vi "解析S2文件.vi"() -> ()   [LabVIEW 2017]
panel:
  out "段地址":u32[](array[numeric]) format="%6x"
  out "输出数组-第一行":i32[][](array[numeric]) format="%02x"
  out "发送数据组":u32[][][](array[numeric]) format="%02x"
  out "数组头-每段":u32[][](array[numeric]) format="%x"
  out "连续数组-中-每小块":u32[][][](array[numeric]) format="%02x"
  out "数据数组2":u32[][](array[numeric]) format="%02x"
  out "地址有间隔":i32[](array[numeric])
  out "段数":i32
  out "数据数组":string[](array[string])
  out "每行字符数":i32[](array[numeric])
  out "地址数组":u32[](array[numeric]) format="%06x"
  in  "停止":bool
  out "行数":i32
  out "数组":string[](array[string])
  # "段尾"
  # "行数"
  # "每行字符"
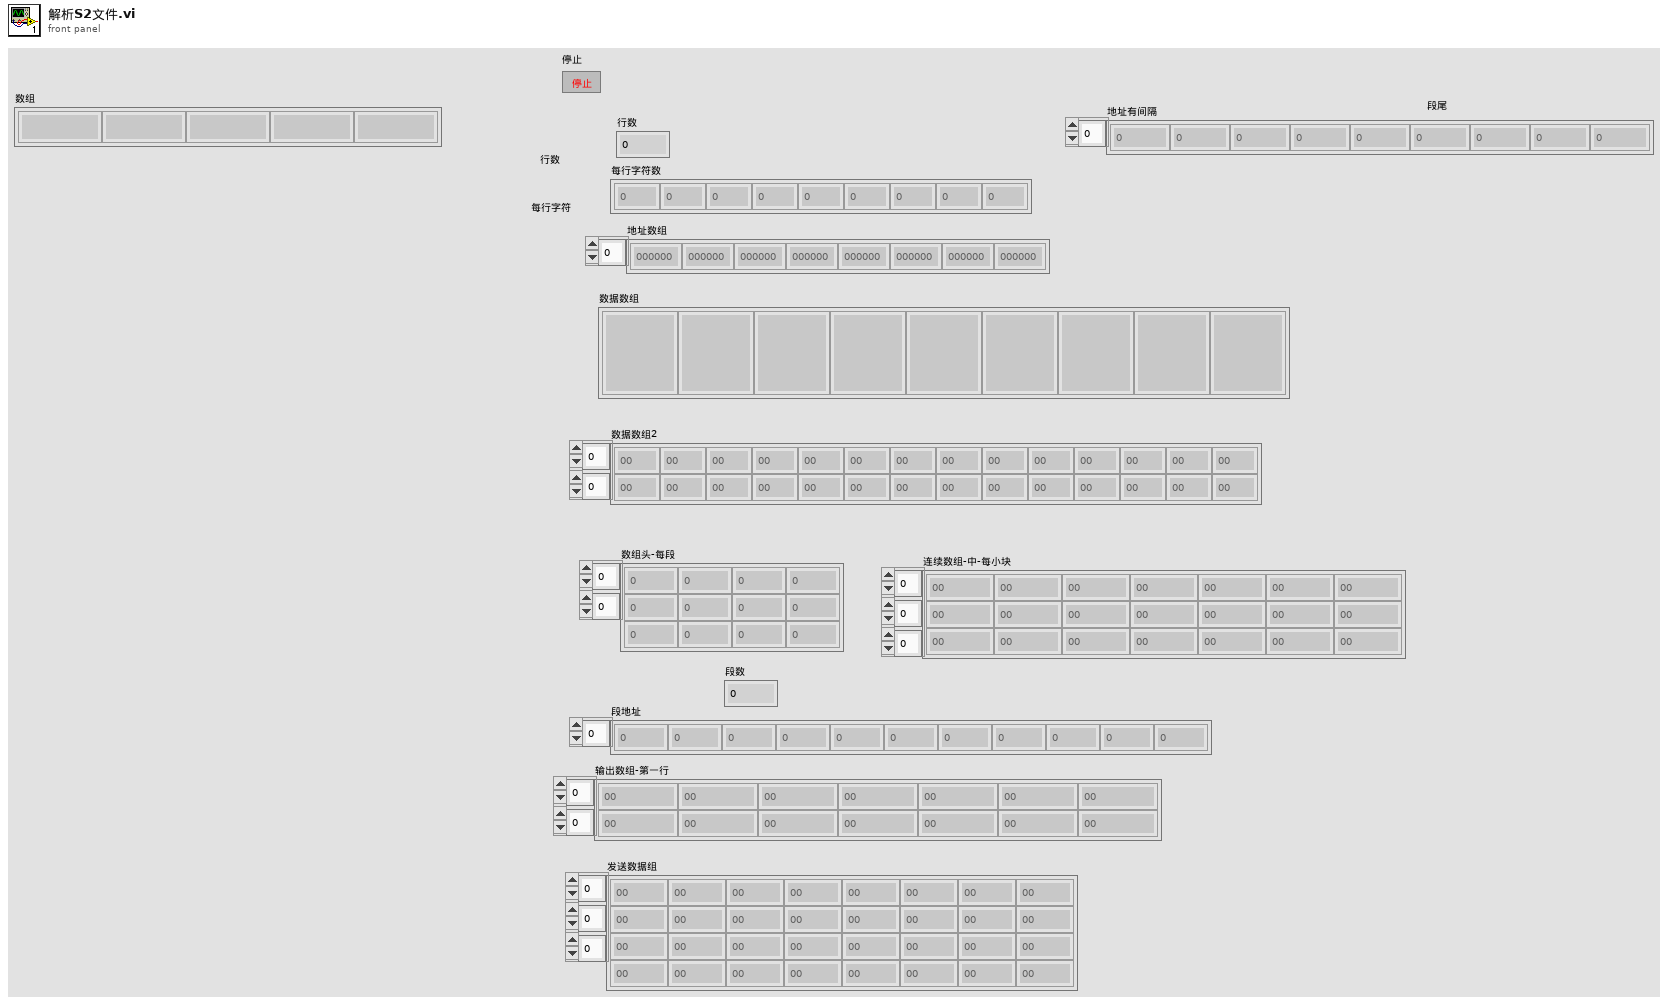
[diagram p1: front panel]
types:
  T1 = enum16{"open", "replace", "create", "open or create", "replace or create", "replace or create with confirmation"}
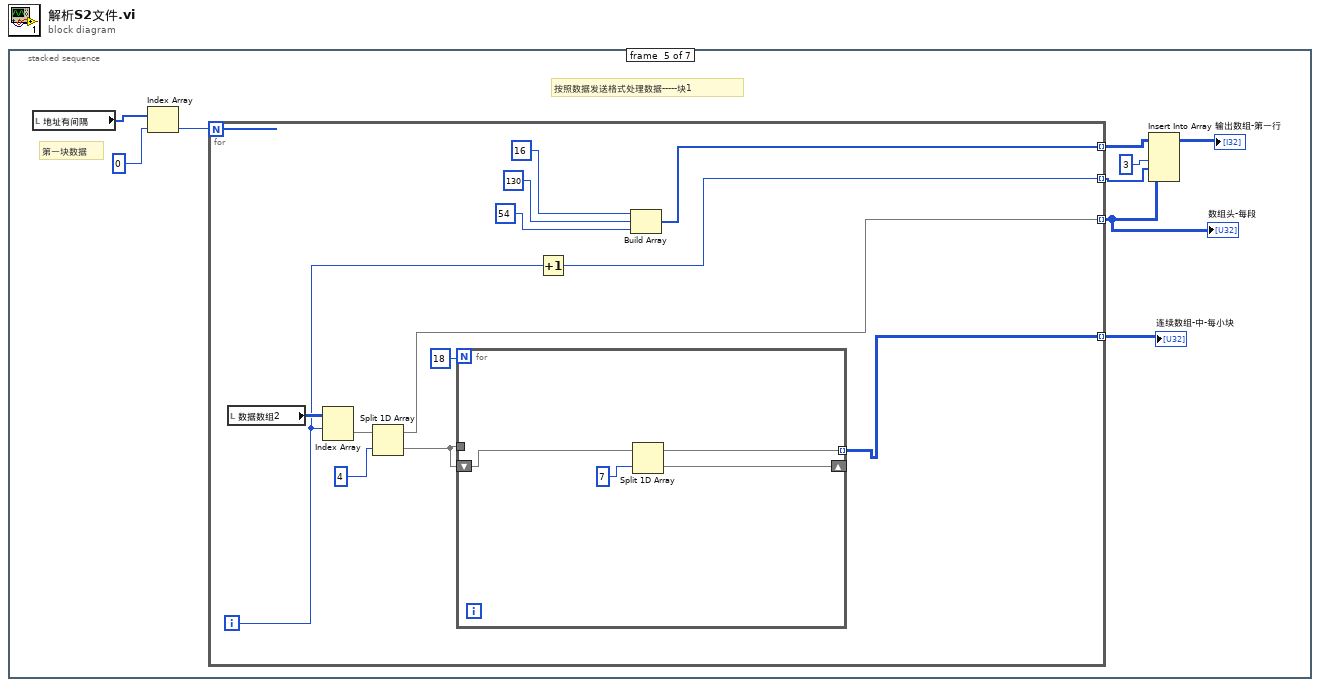
[diagram p0: block diagram]
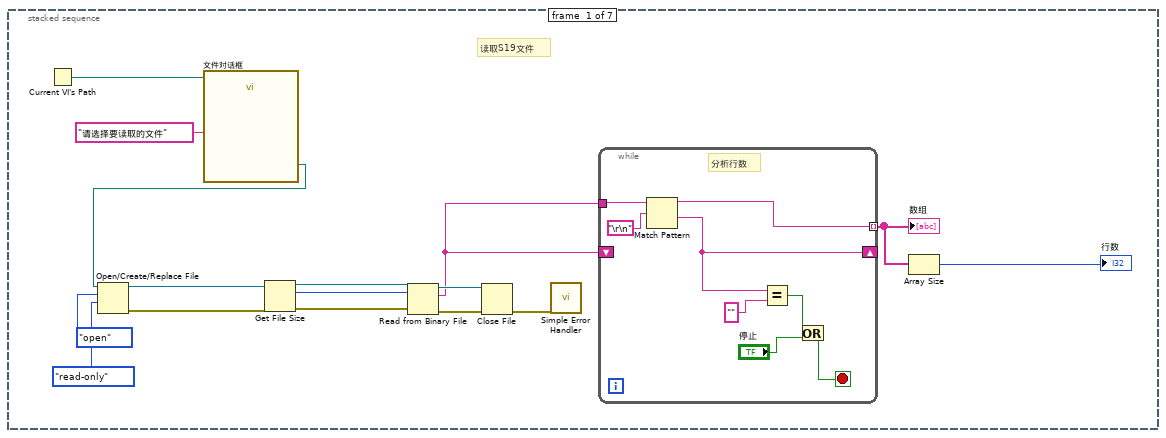
[diagram p2: hidden frame]
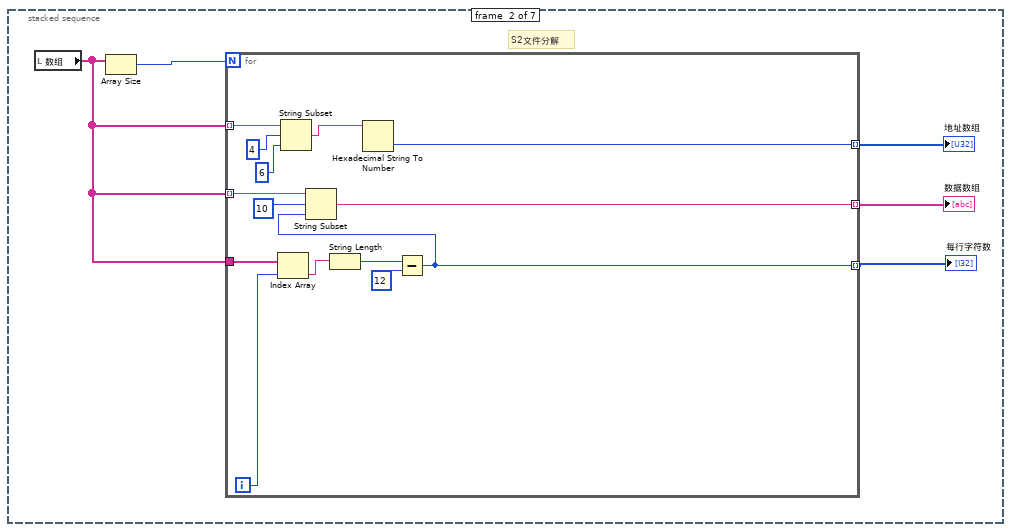
[diagram p3: hidden frame]
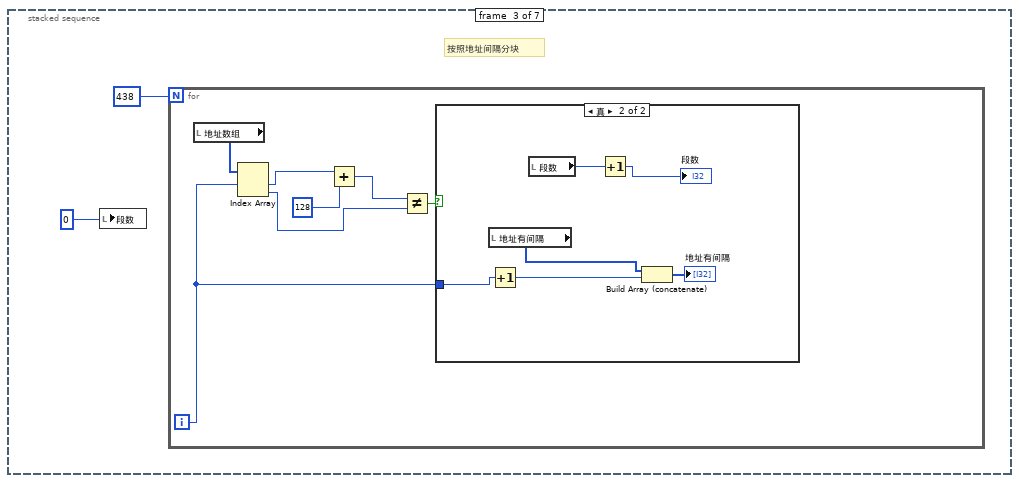
[diagram p4: hidden frame]
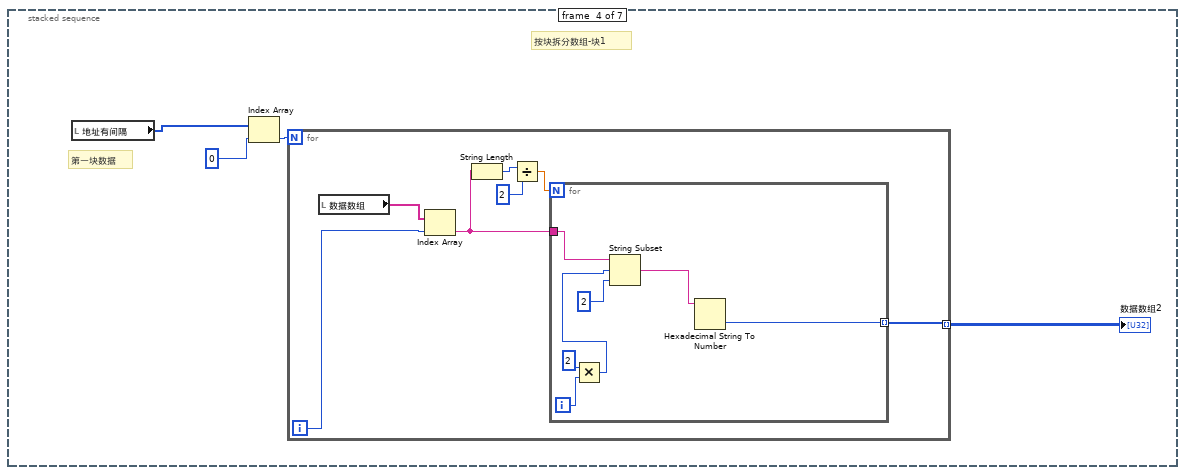
[diagram p6: hidden frame]
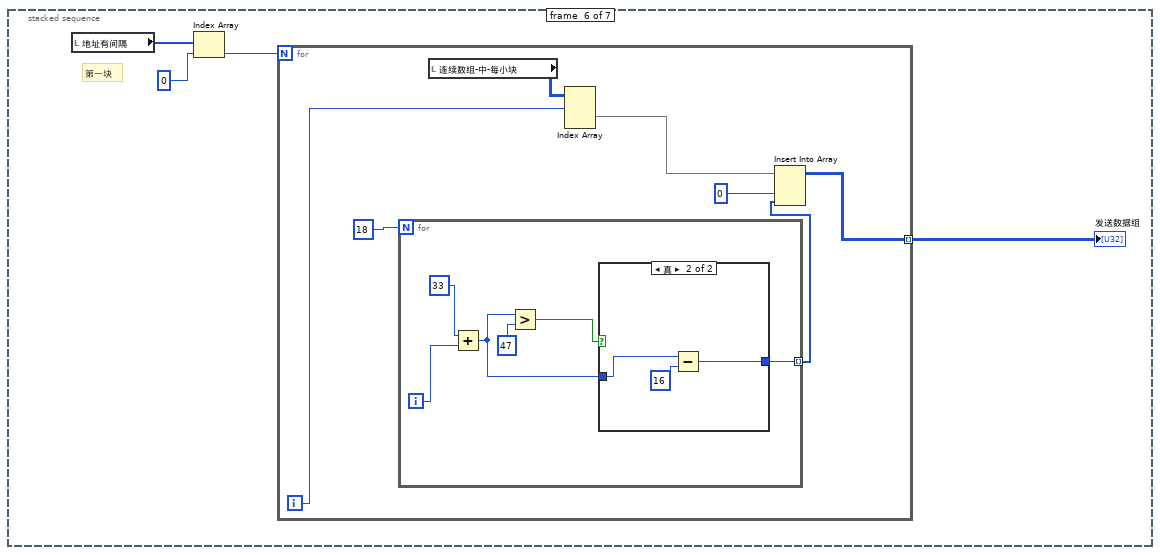
[diagram p7: hidden frame]
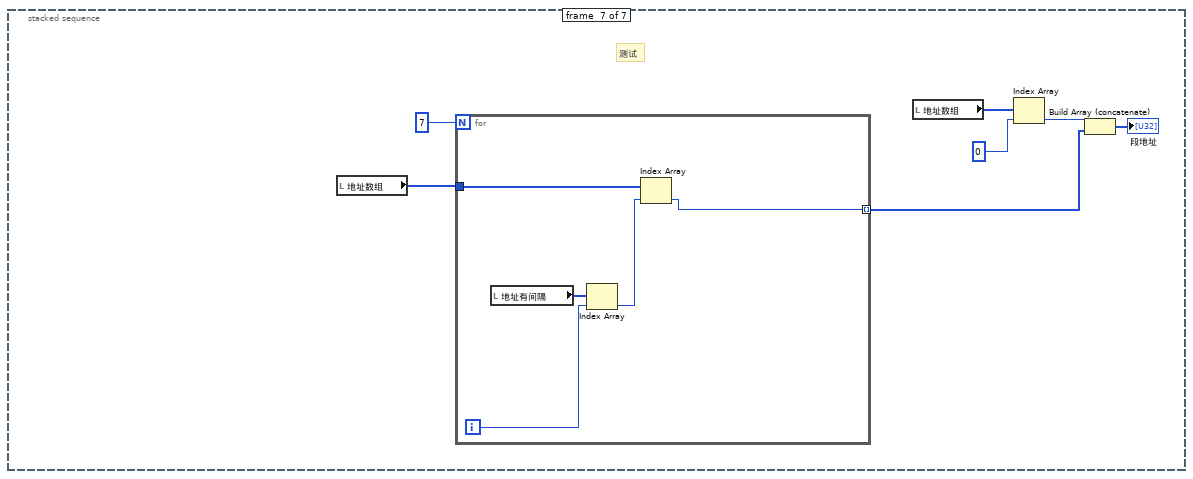
[diagram p9: hidden frame]
diagram:
  n1 = stacked-sequence {
    frame #0 {
      # "读取S19文件"
      n2 = Current VI's Path() -> (path=w5:path)
      n3 = call "文件对话框"("start path"=w5, "prompt"="请选择要读取的文件") -> ("selected path"=w15:path)  [unwired: 10 in, 3 out]
      n4 = Open/Create/Replace File(file path (use dialog)=w15, operation (0:open)=T1."open", access (0:read/write)=enum16{"read/write", "read-only", "write-only"}."read-only") -> (refnum out=w6:refnum<file>, error out=w11:errorcluster)  [unwired: 3 in, 1 out]
      n5 = Get File Size(file=w6, error in=w11) -> (refnum out=w14:refnum<file>, size (in bytes)=w7:i64, 0:w10:errorcluster)
      n6 = Read from Binary File(8:w10, 10:w7, 11:w14) -> (0:w9:errorcluster, 2:w2:string, 3:w16:refnum<file>)  [unwired: 3 in, 1 out]
      n7 = Close File(refnum=w16, error in=w9) -> (error out=w8:errorcluster)  [unwired: 1 out]
      n8 = call <vilib>:"Simple Error Handler.vi"("error in (no error)"=w8) -> ()  [unwired: 4 in, 5 out]
      n9 = while "While循环" {
        tunnel: w2 -> [_]
        tunnel: [w19] -> w1 mode=indexing
        shift-right: [w18] -> _
        shift-left: w2 -> [w17]
        stop <- w22 stop-if-true
        # "分析行数"
        n10 = Match Pattern(string=w17, regular expression="\r\n") -> (before substring=w19:string, after substring=w18:string)  [unwired: 1 in, 2 out]
        n11 = Equal?(x=w18, y="") -> (x = y?=w23:bool)
        n12 = Or(x=w23, y="停止") -> (x .or. y?=w22:bool)
      }
      "数组" <- w1
      n13 = Array Size(array=w1) -> (size(s)=→"行数":i32)
    }
    frame #1 {
      # "S2文件分解"
      n14 = local read "数组"() -> (w27:string[])
      n15 = Array Size(array=w27) -> (size(s)=w25:i32)
      n16 = for {
        N: w25 -> [_]
        tunnel: w27 -> [w43] mode=indexing
        tunnel: [w39] -> w29 mode=indexing
        tunnel: w27 -> [w31]
        tunnel: [w30] -> w28 mode=indexing
        tunnel: w27 -> [w35] mode=indexing
        tunnel: [w33] -> w26 mode=indexing
        i -> [w32]
        n17 = Index Array(array=w31, index=w32) -> (element=w38:string)
        n18 = String Subset(string=w43, offset (0)=4, length (rest)=6) -> (substring=w40:string)
        n19 = String Length(string=w38) -> (length=w37:i32)
        n20 = Hexadecimal String To Number(string=w40) -> (number=w39:u32)  [unwired: 2 in, 1 out]
        n21 = Subtract(x=w37, y=12) -> (x-y=w30:i32)
        n22 = String Subset(string=w35, offset (0)=10, length (rest)=w30) -> (substring=w33:string)
      }
      "地址数组" <- w29
      "每行字符数" <- w28
      "数据数组" <- w26
    }
    frame #2 {
      # "按照地址间隔分块"
      n23 = local write "段数"(0) -> ()
      n24 = for {
        N: 438 -> [_]
        i -> [w49]
        n25 = local read "地址数组"() -> (w50:u32[])
        n26 = Index Array(array=w50, index #1=w49) -> (element #1=w51:u32, element #2=w46:u32)  [unwired: 1 in]
        n27 = Add(x=w51, y=u32 128) -> (x+y=w47:u32)
        n28 = Not Equal?(x=w47, y=w46) -> (x != y?=w48:bool)
        n29 = case shown="真" w48 {
          tunnel: w49 -> [_ w54]
          frame False {
          }
          frame True {
            n30 = local read "地址有间隔"() -> (w55:i32[])
            n31 = Increment(x=w54) -> (x+1=w53:i32)
            n32 = local read "段数"() -> (w58:i32)
            n33 = Increment(x=w58) -> (x+1=→"段数":i32)
            n34 = Build Array (concatenate)(w55, w53) -> (→"地址有间隔":i32[])
          }
        }
      }
    }
    frame #3 {
      # "第一块数据"
      # "按块拆分数组-块1"
      n35 = local read "地址有间隔"() -> (w60:i32[])
      n36 = Index Array(array=w60, index=0) -> (element=w61:i32)
      n37 = for {
        N: w61 -> [_]
        tunnel: [w64] -> w62 mode=indexing
        i -> [w63]
        n38 = local read "数据数组"() -> (w66:string[])
        n39 = Index Array(array=w66, index=w63) -> (element=w67:string)
        n40 = String Length(string=w67) -> (length=w68:i32)
        n41 = Divide(x=w68, y=2) -> (x/y=w69:dbl)
        n42 = for {
          N: w69 -> [_]
          tunnel: w67 -> [w76]
          tunnel: [w74] -> w64 mode=indexing
          i -> [w73]
          n43 = Multiply(x=2, y=w73) -> (x*y=w72:i32)
          n44 = String Subset(string=w76, offset (0)=w72, length (rest)=2) -> (substring=w75:string)
          n45 = Hexadecimal String To Number(string=w75) -> (number=w74:u32)  [unwired: 2 in, 1 out]
        }
      }
      "数据数组2" <- w62
    }
    frame #4 {
      # "第一块数据"
      # "按照数据发送格式处理数据-----块1"
      n46 = local read "地址有间隔"() -> (w85:i32[])
      n47 = Index Array(array=w85, index=0) -> (element=w83:i32)
      n48 = for {
        N: w83 -> [_]
        tunnel: [w93] -> w82 mode=indexing
        tunnel: [w92] -> w77 mode=indexing
        tunnel: [w87] -> w81 mode=indexing
        tunnel: [w86] -> w80 mode=indexing
        i -> [w88]
        n49 = local read "数据数组2"() -> (w98:u32[][])
        n50 = Index Array(array=w98, index (row)=w88) -> (element=w97:u32[])  [unwired: 1 in]
        n51 = Split 1D Array(array=w97, index=4) -> (first subarray=w92:u32[], second subarray=w94:u32[])
        n52 = for {
          N: 18 -> [_]
          tunnel: w94 -> [_]
          tunnel: [w102] -> w93 mode=indexing
          shift-right: [w101] -> _
          shift-left: w94 -> [w99]
          n53 = Split 1D Array(array=w99, index=7) -> (first subarray=w102:u32[], second subarray=w101:u32[])
        }
        n54 = Increment(x=w88) -> (x+1=w86:i32)
        n55 = Build Array(16, 130, 54) -> (w87:i32[])
      }
      "连续数组-中-每小块" <- w82
      "数组头-每段" <- w77
      n56 = Insert Into Array(array=w81, index (col)=3, new element #1=w80, new element #2=w77) -> (→"输出数组-第一行":i32[][])  [unwired: 1 in]
    }
    frame #5 {
      # "第一块"
      n57 = local read "地址有间隔"() -> (w103:i32[])
      n58 = Index Array(array=w103, index=0) -> (element=w105:i32)
      n59 = for {
        N: w105 -> [_]
        tunnel: [w107] -> w104 mode=indexing
        i -> [w108]
        n60 = for {
          N: 18 -> [_]
          tunnel: [w114] -> w109 mode=indexing
          i -> [w118]
          n61 = Add(x=33, y=w118) -> (x+y=w115:i32)
          n62 = Greater?(x=w115, y=47) -> (0:w116:bool)
          n63 = case shown="真" w116 {
            tunnel: w115 -> [w120 w123]
            tunnel: [w120 w122] -> w114
            frame False {
            }
            frame True {
              n64 = Subtract(x=w123, y=16) -> (x-y=w122:i32)
            }
          }
        }
        n65 = local read "连续数组-中-每小块"() -> (w113:u32[][][])
        n66 = Index Array(array=w113, index (dim 0)=w108) -> (element=w112:u32[][])  [unwired: 2 in]
        n67 = Insert Into Array(array=w112, index (col)=0, new element=w109) -> (w107:u32[][])  [unwired: 1 in]
      }
      "发送数据组" <- w104
    }
    frame #6 {
      # "测试"
      n68 = local read "地址数组"() -> (w130:u32[])
      n69 = for {
        N: 7 -> [_]
        tunnel: w130 -> [w132]
        tunnel: [w131] -> w125 mode=indexing
        i -> [w134]
        n70 = local read "地址有间隔"() -> (w135:i32[])
        n71 = Index Array(array=w135, index=w134) -> (element=w133:i32)
        n72 = Index Array(array=w132, index=w133) -> (element=w131:u32)
      }
      n73 = local read "地址数组"() -> (w127:u32[])
      n74 = Index Array(array=w127, index=0) -> (element=w126:u32)
      n75 = Build Array (concatenate)(w126, w125) -> (→"段地址":u32[])
    }
  }
